vi "Initialize Hardware References.vi"(8 "error in (no error)":errorcluster, 10 "UI":refnum<queue>, 11 "Hardware Resources in":T1) -> (0 "error out":errorcluster, 3 "Hardware Resources out":T1)   [LabVIEW 2014, in "AvaSpec.lvlib" / "AvaSpec Acquisition.lvlib"]
doc: "Initialize the hardware references."
uses:
  AvaSpec Acquisition.lvlib
  Hardware Configuration.ctl
  Libraries/AS-5216-DLL/AVS settings.ctl
  Sphere Indicator.ctl
  Settings/Measurement Type.ctl
  support/Message Queue/Message Cluster.ctl
  support/Message Queue/Enqueue Message (Single).vi
  Libraries/AS-5216-DLL/Avantes Spectrometer Functions.lvlib
  support/Message Queue/AvaSpec Message Queue.lvlib
  AvaSpec.lvlib
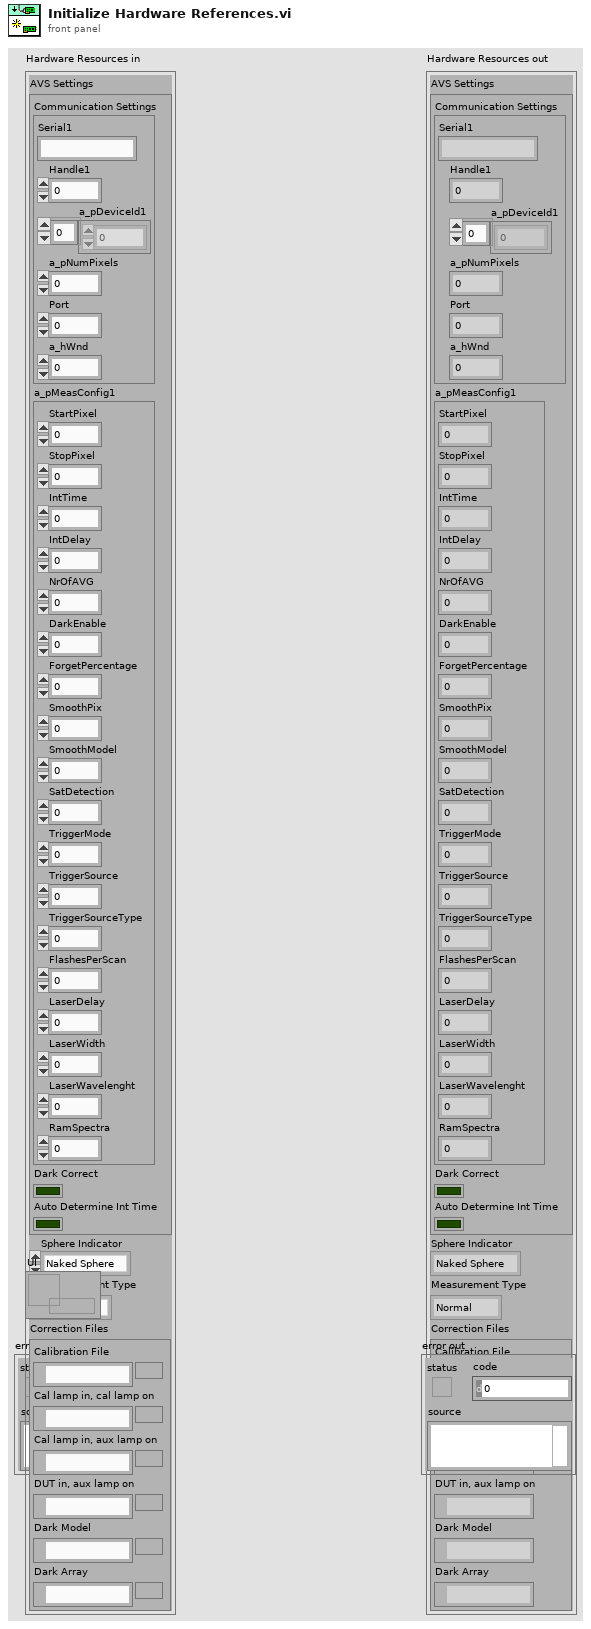
[diagram p1: front panel]
types:
  T1 = typedef "AvaSpec.lvlib/AvaSpec Acquisition.lvlib/Hardware Configuration.ctl" = cluster{"AVS Settings":T2, "Sphere Indicator":T3, "Measurement Type":T4, "Correction Files":cluster{"Calibration File":path, "Cal lamp in, cal lamp on":path, "Cal lamp in, aux lamp on":path, "DUT in, aux lamp on":path, "Dark Model":path, "Dark Array":path}}
  T2 = typedef "AvaSpec.lvlib/AVS settings.ctl" = cluster{"Communication Settings":cluster{"Serial1":string, "Handle1":i32, "a_pDeviceId1":u8[], "a_pNumPixels":u16, "Port":i32, "a_hWnd":i32}, "a_pMeasConfig1":cluster{"StartPixel":u16, "StopPixel":u16, "IntTime":sgl, "IntDelay":u32, "NrOfAVG":u32, "DarkEnable":u8, "ForgetPercentage":u8, "SmoothPix":u16, "SmoothModel":u8, "SatDetection":u8, "TriggerMode":u8, "TriggerSource":u8, "TriggerSourceType":u8, "FlashesPerScan":u16, "LaserDelay":u32, "LaserWidth":u32, "LaserWavelenght":sgl, "RamSpectra":u16}, "Dark Correct":bool, "Auto Determine Int Time":bool}
  T3 = typedef "AvaSpec.lvlib/Sphere Indicator.ctl" = enum16{"Naked Sphere", "Insulated Sphere"}
  T4 = typedef "AvaSpec.lvlib/AvaSpec Acquisition.lvlib/Measurement Type.ctl" = enum16{"Normal", "Calibration", "Dark"}
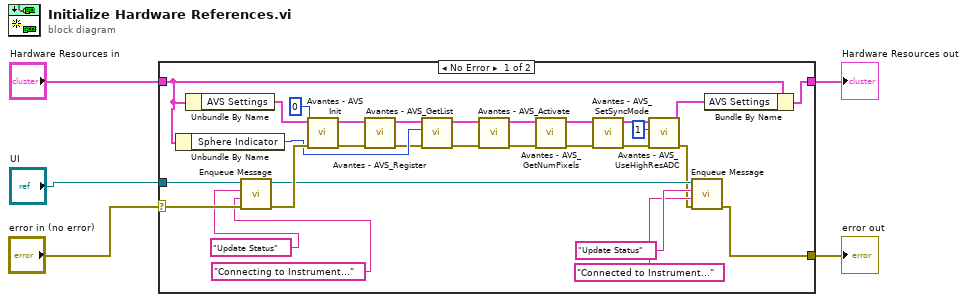
[diagram p0: block diagram]
diagram:
  n1 = case shown="No Error" "error in (no error)" {
    selector: "error in (no error)" -> [w30 w35]
    tunnel: [w23 w35] -> w4
    tunnel: "Hardware Resources in" -> [w18 w36]
    tunnel: [w19 w36] -> w2
    tunnel: "UI" -> [w31 _]
    frame No Error {
      n2 = Unbundle By Name(w18) -> ("Sphere Indicator"=w17:T3)
      n3 = Unbundle By Name(w18) -> ("AVS Settings"=w22:T2)
      n4 = call-poly "Enqueue Message.vi"("error in (no error)"=w30, "Message Data"="Connecting to Instrument..." ("Message"), "Message"="Update Status", "Message Queue"=w31) -> ("error out"=w29:errorcluster, "dup Message Queue"=w26:refnum<queue>)  [unwired: 6 in]
      n5 = call "Avantes - AVS Init.vi"("error in (no error)"=w29, "a_Port"=0, "AVS Settings In"=w22) -> ("error out"=w32:errorcluster, "AVS Settings Out"=w33:T2)  [unwired: 7 in]
      n6 = call "Avantes - AVS_Register.vi"("error in (no error)"=w32, "AVS Settings In"=w33) -> ("error out"=w15:errorcluster, "AVS Settings Out"=w16:T2)  [unwired: 8 in]
      n7 = call "Avantes - AVS_GetList.vi"("error in (no error)"=w15, "Sphere Indicator"=w17, "AVS Settings In"=w16) -> ("error out"=w9:errorcluster, "AVS Settings Out"=w14:T2)  [unwired: 7 in]
      n8 = call "Avantes - AVS_Activate.vi"("error in (no error)"=w9, "AVS Settings In"=w14) -> ("error out"=w10:errorcluster, "AVS Settings Out"=w13:T2)  [unwired: 8 in]
      n9 = call "Avantes - AVS_GetNumPixels.vi"("error in (no error)"=w10, "AVS Settings In"=w13) -> ("error out"=w11:errorcluster, "AVS Settings Out"=w12:T2)  [unwired: 8 in]
      n10 = call "Avantes - AVS_SetSyncMode.vi"("error in (no error)"=w11, "AVS Settings In"=w12) -> ("error out"=w8:errorcluster, "AVS Settings Out"=w7:T2)  [unwired: 8 in]
      n11 = call "Avantes - AVS_UseHighResADC.vi"("error in (no error)"=w8, "a_Enable"=u8 1, "AVS Settings In"=w7) -> ("error out"=w21:errorcluster, "AVS Settings Out"=w20:T2)  [unwired: 7 in]
      n12 = call-poly "Enqueue Message.vi"("error in (no error)"=w21, "Message Data"="Connected to Instrument..." ("Message"), "Message"="Update Status", "Message Queue"=w26) -> ("error out"=w23:errorcluster)  [unwired: 6 in, 1 out]
      n13 = Bundle By Name(cluster=w18, "AVS Settings"=w20) -> (w19:T1)
    }
    frame Error {
    }
  }
  "Hardware Resources out" <- w2
  "error out" <- w4
